vi "Test - Firmware Revision.vi"(8 "error in (no error)":errorcluster) -> (0 "error out":errorcluster)   [LabVIEW 2020]
uses:
  Library - Test Executive.llb/Test Executive.lvlib
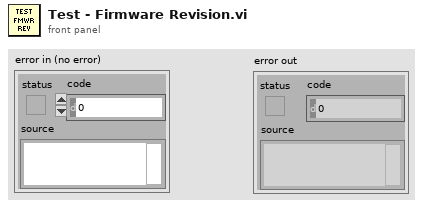
[diagram p1: front panel]
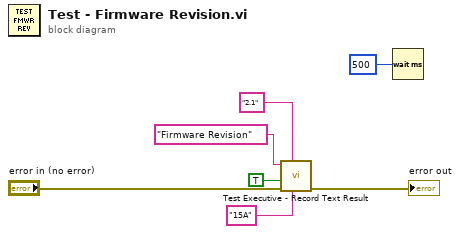
[diagram p0: block diagram]
diagram:
  n1 = call "Test Executive - Record Text Result.vi"("Text"="15A", "Test Ref"="2.1", "error in (no error)"="error in (no error)", "Pass"=TRUE, "Test Name"="Firmware Revision") -> ("error out"=→"error out":errorcluster)  [unwired: 6 in]
  n2 = Wait (ms)(milliseconds to wait=u32 500) -> ()  [unwired: 1 out]
